vi "NicmosGetTemperature.vi"(9 "error in (no error)":errorcluster caption="error out (no error)") -> (2 "Temperature graph":cluster{"T1":dbl, "T2":dbl}(graph)={"T1"=79.0, "T2"=111.7}, 6 "error out":errorcluster)   [LabVIEW 2009]
uses:
  Controls/NICMOS.COMMAND.ctl
  Controls/NICMOS.COMMANDBASIC.ctl
  Controls/NICMOS.READOUT.ctl
  Controls/NICMOS.FILTERCOMMAND.ctl
  Controls/NICMOS.FILTER.ctl
  Controls/NICMOS.TEMPERATURE.ctl
panel:
  # "To run continuously!!!"
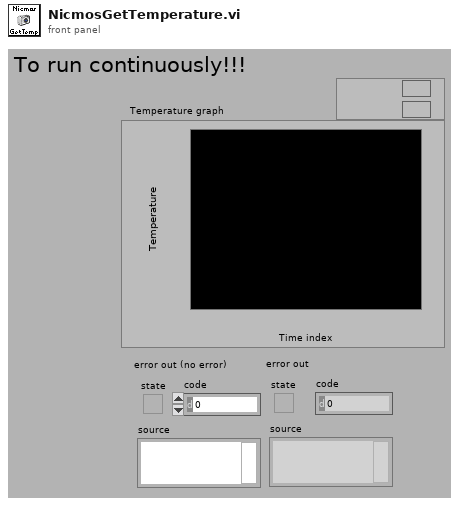
[diagram p1: front panel]
types:
  T1 = typedef "NICMOS.TEMPERATURE.ctl" = cluster{"T1":dbl, "T2":dbl}
  T2 = typedef "NICMOS.COMMAND.ctl" = cluster{"Command":T3, "READOUT":T4, "FILTERCOMMAND":T5, "ACQUISITION":i32, "Done":refnum<k4>}
  T3 = typedef "NICMOS.COMMANDBASIC.ctl" = enum16{"WRITE BANKS", "SET FILTER", "HOME FILTER", "QUERY TEMP", "CONFIGURE", "START", "ACQUISITION", "STOP", "QUIT"}
  T4 = typedef "NICMOS.READOUT.ctl" = cluster{"Readout":i32, "Deglitch":i32, "Framerate":dbl[unit], "Bank":i32}
  T5 = typedef "NICMOS.FILTERCOMMAND.ctl" = cluster{"FILTER":T6, "INIT":bool}
  T6 = typedef "NICMOS.FILTER.ctl" = string
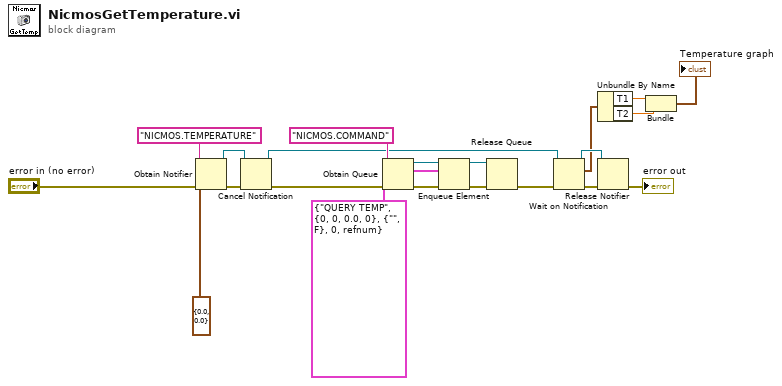
[diagram p0: block diagram]
diagram:
  w12 = T2 {"Command"=enum."QUERY TEMP", "READOUT"={"Readout"=0, "Deglitch"=0, "Framerate"=0.0, "Bank"=0}, "FILTERCOMMAND"={"FILTER"="", "INIT"=FALSE}, "ACQUISITION"=0, "Done"=refnum} ("NicmosCommand")
  n1 = Obtain Notifier(name (unnamed)="NICMOS.TEMPERATURE" ("nom (aucun)"), notification data type=T1 {"T1"=0.0, "T2"=0.0} ("Nicmos Status"), error in (no error)="error in (no error)") -> (notifier out=w5:refnum<notifier>, error out=w6:errorcluster)  [unwired: 1 in, 1 out]
  n2 = Cancel Notification(0:w5, 3:w6) -> (8:w4:refnum<notifier>, 11:w2:errorcluster)  [unwired: 1 out]
  n3 = Obtain Queue(name (unnamed)="NICMOS.COMMAND" ("nom (aucun)"), element data type=w12, error in (no error)=w2) -> (queue out=w10:refnum<queue>, error out=w1:errorcluster)  [unwired: 2 in, 1 out]
  n4 = Enqueue Element(queue=w10, element=w12, error in (no error)=w1) -> (queue out=w9:refnum<queue>, error out=w21:errorcluster)  [unwired: 1 in, 1 out]
  n5 = Release Queue(queue=w9, error in (no error)=w21) -> (error out=w11:errorcluster)  [unwired: 1 in, 2 out]
  n6 = Wait on Notification(notifier=w4, error in (no error)=w11) -> (notifier out=w8:refnum<notifier>, notification=w7:T1, error out=w16:errorcluster)  [unwired: 2 in, 1 out]
  n7 = Unbundle By Name(w7) -> ("T1"=w15:dbl, "T2"=w14:dbl)
  n8 = Release Notifier(notifier=w8, error in (no error)=w16) -> (error out=→"error out":errorcluster)  [unwired: 1 in, 2 out]
  n9 = Bundle("T1"=w15, "T2"=w14) -> (→"Temperature graph":cluster{"T1":dbl, "T2":dbl})  [unwired: 1 in]
